vi "Get Node Attributes.vi"(8 "error in (no error)":errorcluster, 9 "Attributes Cluster":variant, 10 "Node Name (exact)":string="//rect", 11 "ParseSVG in":refnum<class "ParseSVG.lvclass">) -> (0 "error out":errorcluster, 1 "[Attributes Cluster]":variant[](array[variant]), 2 "Positions":i32[](array[numeric]), 3 "ParseSVG out":refnum<class "ParseSVG.lvclass">)   [LabVIEW 2019, in "ParseSVG.lvclass"]
uses:
  ParseSVG.lvclass
  ParseSVG.lvclass/ParseSVG.ctl
  <vilib>/xml/NI_XML.lvlib
  <vilib>/xml/Close Reference(Node).vi
  <resource>/objmgr/DOMUserDefRef.rc
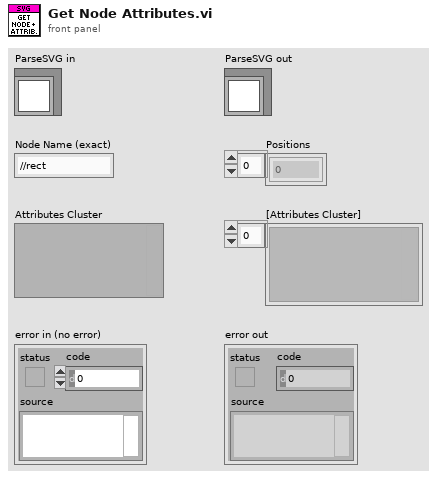
[diagram p1: front panel]
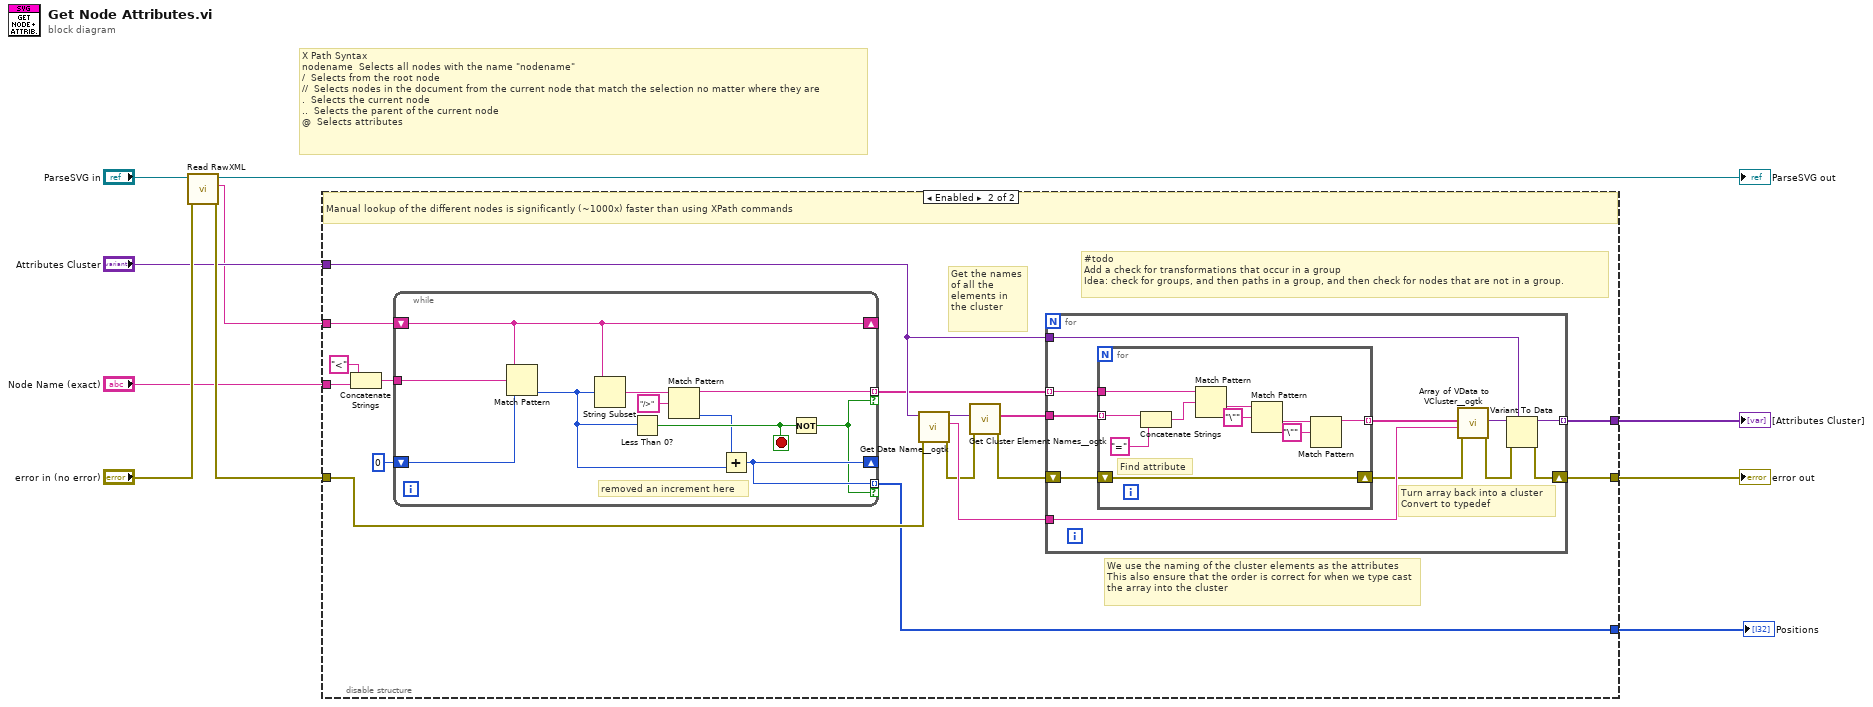
[diagram p0: block diagram]
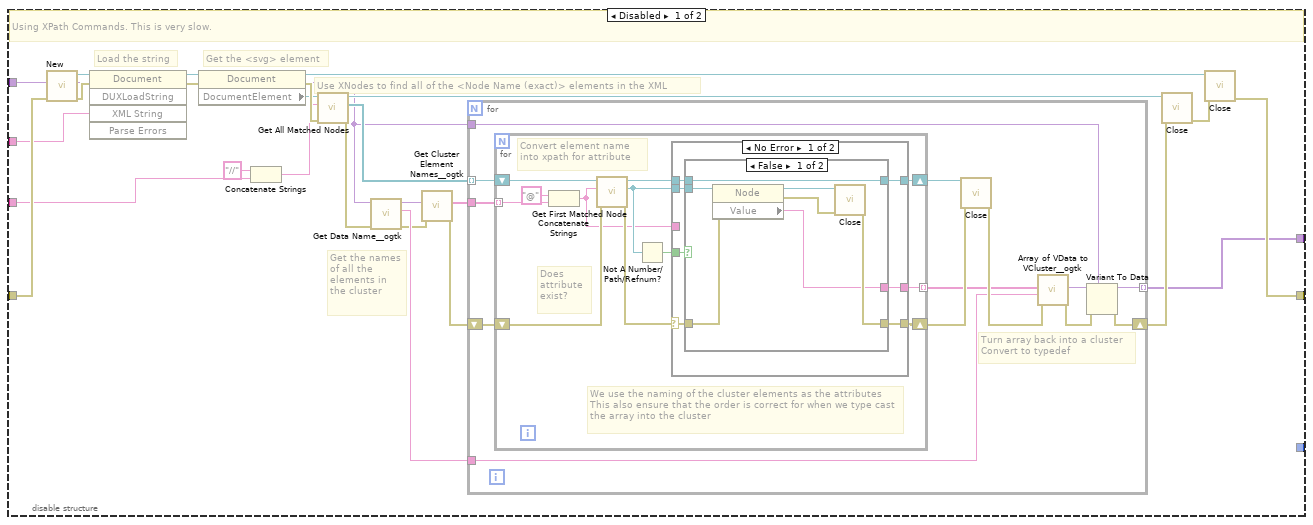
[diagram p2: hidden frame]
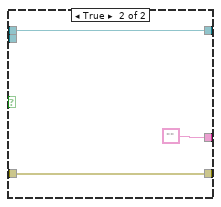
[diagram p3: hidden frame]
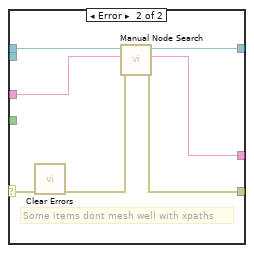
[diagram p4: hidden frame]
diagram:
  # "X Path Syntax\nnodename \tSelects all nodes with the name \"nodename\"\n/ \tSelects from the root node\n// \tSelects nodes in the document from the current node that match the selection no matter where they are\n. \tSelects the current node\n.. \tSelects the parent of the current node\n@ \tSelects attributes"
  n1 = call "Read RawXML.vi"("error in (no error)"="error in (no error)", "ParseXML in"="ParseSVG in") -> ("error out"=w8:errorcluster, "RawXML"=w2:string, "ParseXML out"=→"ParseSVG out":refnum<class "ParseSVG.lvclass">)  [unwired: 7 in]
  n2 = disable-structure shown="Enabled" {
    disable-tunnel: [w34 w94] -> w9
    disable-tunnel: w8 -> [w33 w86]
    disable-tunnel: "Node Name (exact)" -> [w20 w88]
    disable-tunnel: [w17 w95] -> w4
    disable-tunnel: "Attributes Cluster" -> [w16 w96]
    disable-tunnel: w2 -> [w15 w89]
    disable-tunnel: [_ w85] -> w1
    frame Disabled {
      # "Get the names of all the elements in the cluster"
      # "Use XNodes to find all of the <Node Name (exact)> elements in the XML"
      # "Get the <svg> element"
      # "Load the string"
      # "Using XPath Commands. This is very slow."
      n3 = call <vilib>:"New.vi"("error in (no error)"=w33) -> ("error out"=w32:errorcluster, "DOM document out"=w27:refnum<k20>)  [unwired: 7 in]
      n4 = invoke class="Document" method="DUXLoadString"(reference=w27, error in=w32, "XML String"=w15) -> (reference out=w26:refnum<k20>, error out=w31:errorcluster)  [unwired: 2 in, 3 out]
      n5 = property class="Document"(reference=w26, error in=w31) -> (reference out=w25:refnum<k20>, error out=w30:errorcluster, "DocumentElement"=w24:refnum<k20>)
      n6 = Concatenate Strings("//" ("string"), w20) -> (w19:string)
      n7 = call <vilib>:"Get All Matched Nodes.vi"("error in (no error)"=w30, "XPath expression"=w19, "node in"=w24) -> ("error out"=w29:errorcluster, "node result array"=w22:refnum<k20>[], "node out"=w23:refnum<k20>)  [unwired: 6 in]
      n8 = call <userlib>:"Get Data Name__ogtk.vi"("error in (no error)"=w29, "Data"=w16) -> ("error out"=w11:errorcluster, "Data Name"=w21:string, "Data dup"=w14:variant)  [unwired: 7 in]
      n9 = call <userlib>:"Get Cluster Element Names__ogtk.vi"("error in (no error)"=w11, "Cluster"=w14) -> ("error out"=w12:errorcluster, "Element Names"=w13:string[])  [unwired: 8 in]
      n10 = for {
        tunnel: w22 -> [w43] mode=indexing
        shift-right: [w45] -> w35
        shift-left: w12 -> [w44]
        tunnel: [w41] -> w17 mode=indexing
        tunnel: w13 -> [w38]
        tunnel: w21 -> [w37]
        tunnel: w16 -> [w36]
        # "Turn array back into a cluster\nConvert to typedef"
        n11 = for {
          shift-right: [w59] -> w48
          shift-left: w44 -> [w60]
          shift-right: [w53] -> w42
          shift-left: w43 -> [w57]
          tunnel: [w50] -> w40 mode=indexing
          tunnel: w38 -> [w51] mode=indexing
          # "Convert element name into xpath for attribute"
          # "Does attribute exist?"
          # "We use the naming of the cluster elements as the attributes\nThis also ensure that the order is correct for when we type cast the array into the cluster"
          n12 = Concatenate Strings("@" ("string"), w51) -> (w49:string)
          n13 = call <vilib>:"Get First Matched Node.vi"("error in (no error)"=w60, "XPath expression"=w49, "node in"=w57) -> ("error out"=w58:errorcluster, "node result"=w56:refnum<k20>, "node out"=w54:refnum<k20>)  [unwired: 6 in]
          n14 = Not A Number/Path/Refnum?(number/path/refnum=w56) -> (NaN/Path/Refnum?=w55:bool)
          n15 = case shown="No Error" w58 {
            selector: w58 -> [w66 w83]
            tunnel: [w67 w84] -> w59
            tunnel: w56 -> [w65 _]
            tunnel: w55 -> [w64 _]
            tunnel: w54 -> [w63 w80]
            tunnel: [w62 w81] -> w53
            tunnel: [w61 w78] -> w50
            tunnel: w49 -> [_ w79]
            frame No Error {
              n16 = case shown="False" w64 {
                tunnel: w66 -> [w74 w77]
                tunnel: [w73 w77] -> w67
                tunnel: w65 -> [w71 _]
                tunnel: w63 -> [w70 w76]
                tunnel: [w70 w76] -> w62
                tunnel: [w69 ""] -> w61
                frame False {
                  n17 = property class="Node"(reference=w71, error in=w74) -> (reference out=w72:refnum<k20>, error out=w68:errorcluster, "Value"=w69:string)
                  n18 = call-poly <vilib>:"Close.vi"("error in (no error)"=w68, "node"=w72) -> ("error out"=w73:errorcluster)  [unwired: 7 in]
                }
                frame True {
                }
              }
            }
            frame Error {
              # "Some items dont mesh well with xpaths"
              n19 = call <vilib>:"Clear Errors.vi"("error in (no error)"=w83) -> ("error out"=w82:errorcluster)  [unwired: 5 in, 1 out]
              n20 = call "Manual Node Search.vi"("error in (no error)"=w82, "XPath Syntax"=w79, "Node in"=w80) -> ("error out"=w84:errorcluster, "Value"=w78:string, "Node out"=w81:refnum<k20>)  [unwired: 6 in]
            }
          }
        }
        n21 = call-poly <vilib>:"Close.vi"("error in (no error)"=w48, "node"=w42) -> ("error out"=w47:errorcluster)  [unwired: 7 in]
        n22 = call <userlib>:"Array of VData to VCluster__ogtk.vi"("error in (no error)"=w47, "Cluster Name"=w37, "Array"=w40) -> ("error out"=w46:errorcluster, "VCluster"=w39:variant)  [unwired: 7 in]
        n23 = Variant To Data(error in=w46, type=w36, Variant=w39) -> (data=w41:variant, error out=w45:errorcluster)
      }
      n24 = call-poly <vilib>:"Close.vi"("error in (no error)"=w35, "node"=w23) -> ("error out"=w28:errorcluster)  [unwired: 7 in]
      n25 = call-poly <vilib>:"Close.vi"("error in (no error)"=w28, "node"=w25) -> ("error out"=w34:errorcluster)  [unwired: 7 in]
    }
    frame Enabled {
      # "#todo\nAdd a check for transformations that occur in a group\nIdea: check for groups, and then paths in a group, and then check for nodes that are not in a group."
      # "We use the naming of the cluster elements as the attributes\nThis also ensure that the order is correct for when we type cast the array into the cluster"
      # "Get the names of all the elements in the cluster"
      # "Manual lookup of the different nodes is significantly (~1000x) faster than using XPath commands"
      n26 = Concatenate Strings("<" ("regular expression"), w88) -> (w87:string)
      n27 = while {
        shift-right: [w111] -> _
        shift-left: w89 -> [w111]
        shift-right: [w103] -> _
        shift-left: 0 -> [w109]
        tunnel: [w107] -> w91 mode=indexing if=w102
        tunnel: [w103] -> w85 mode=indexing if=w102
        tunnel: w87 -> [w101]
        stop <- w106 stop-if-true
        # "removed an increment here"
        n28 = Match Pattern(string=w111, regular expression=w101, offset (0)=w109) -> (offset past match=w104:i32)  [unwired: 3 out]
        n29 = String Subset(string=w111, offset (0)=w104) -> (substring=w110:string)  [unwired: 1 in]
        n30 = Less Than 0?(x=w104) -> (x < 0?=w106:bool)
        n31 = Match Pattern(string=w110, regular expression="/>") -> (before substring=w107:string, offset past match=w105:i32)  [unwired: 1 in, 2 out]
        n32 = Add(x=w105, y=w104) -> (x+y=w103:i32)
        n33 = Not(x=w106) -> (.not. x?=w102:bool)
      }
      n34 = call <userlib>:"Get Data Name__ogtk.vi"("error in (no error)"=w86, "Data"=w96) -> ("error out"=w97:errorcluster, "Data Name"=w100:string, "Data dup"=w99:variant)  [unwired: 7 in]
      n35 = call <userlib>:"Get Cluster Element Names__ogtk.vi"("error in (no error)"=w97, "Cluster"=w99) -> ("error out"=w93:errorcluster, "Element Names"=w98:string[])  [unwired: 8 in]
      n36 = for {
        shift-right: [w121] -> w94
        shift-left: w93 -> [w120]
        tunnel: [w119] -> w95 mode=indexing
        tunnel: w98 -> [w116]
        tunnel: w100 -> [w115]
        tunnel: w96 -> [w114]
        tunnel: w91 -> [w112] mode=indexing
        # "Turn array back into a cluster\nConvert to typedef"
        n37 = for {
          shift-right: [w132] -> w113
          shift-left: w120 -> [w132]
          tunnel: [w126] -> w118 mode=indexing
          tunnel: w116 -> [w124] mode=indexing
          tunnel: w112 -> [w131]
          # "Find attribute"
          n38 = Concatenate Strings(w124, "=" ("string")) -> (w125:string)
          n39 = Match Pattern(string=w131, regular expression=w125) -> (after substring=w130:string)  [unwired: 1 in, 3 out]
          n40 = Match Pattern(string=w130, regular expression="\"") -> (after substring=w128:string)  [unwired: 1 in, 3 out]
          n41 = Match Pattern(string=w128, regular expression="\"") -> (before substring=w126:string)  [unwired: 1 in, 3 out]
        }
        n42 = call <userlib>:"Array of VData to VCluster__ogtk.vi"("error in (no error)"=w113, "Cluster Name"=w115, "Array"=w118) -> ("error out"=w122:errorcluster, "VCluster"=w117:variant)  [unwired: 7 in]
        n43 = Variant To Data(error in=w122, type=w114, Variant=w117) -> (data=w119:variant, error out=w121:errorcluster)
      }
    }
  }
  "error out" <- w9
  "[Attributes Cluster]" <- w4
  "Positions" <- w1
